vi "Scale Image - subvi.vi"(8 "Array Size":i32, 9 "99:1?":bool, 10 "Black/White Levels":cluster{ext, ext}(slide)={1.0, 65535.0} scale=-32768.0..32767.0, 11 "Image Array":i32[][](array[numeric])) -> (2 "Black/White Levels Out":cluster{ext, ext}(slide)={1.0, 65535.0} scale=-32768.0..32767.0, 3 "Image Array 2":i32[][](array[numeric]))   [LabVIEW 2014]
panel:
  out "Min":ext
  out "Max":ext
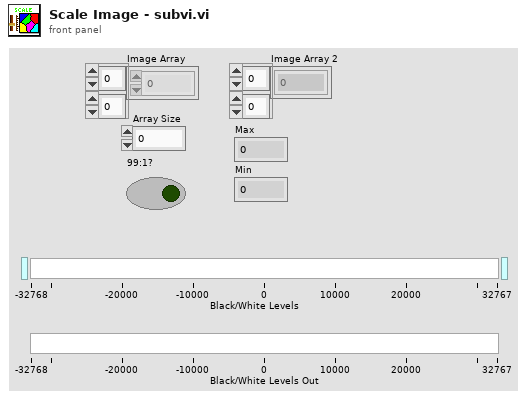
[diagram p1: front panel]
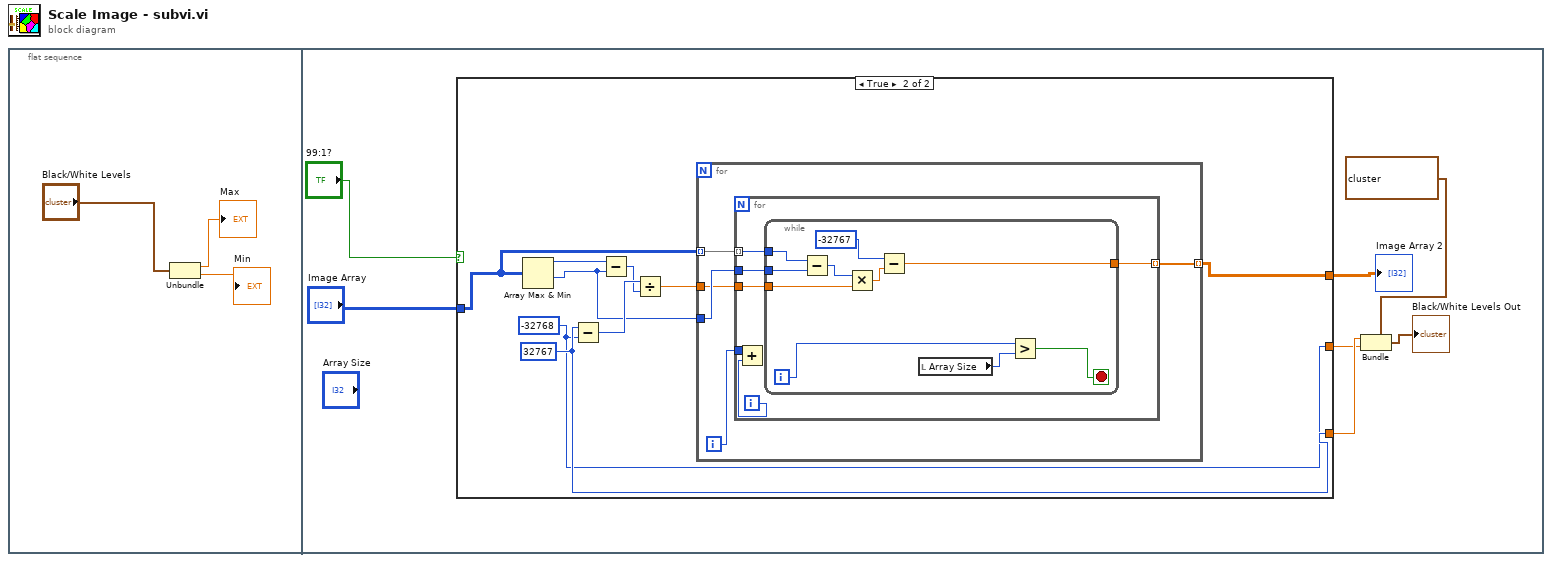
[diagram p0: block diagram]
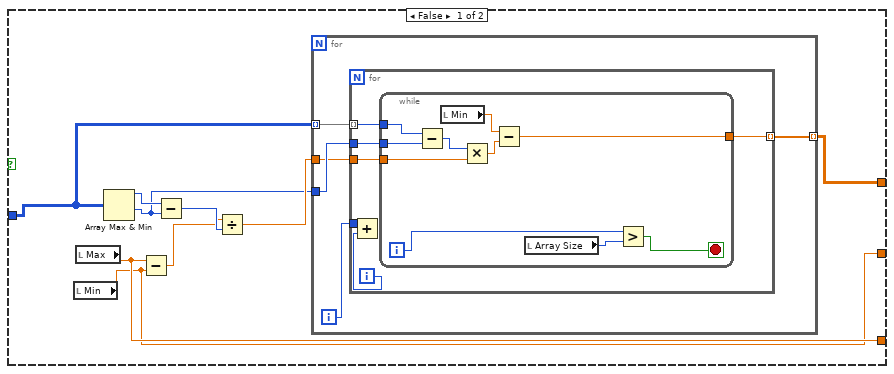
[diagram p2: hidden frame]
diagram:
  n1 = flat-sequence {
    frame #0 {
      n2 = Unbundle("Black/White Levels") -> (→"Max":ext, →"Min":ext)
    }
    frame #1 {
      n3 = case shown="True" "99:1?" {
        tunnel: "Image Array" -> [w16 w43]
        tunnel: [w14 w44] -> w10
        tunnel: [w12 w42] -> w5
        tunnel: [w11 w41] -> w4
        frame False {
          n4 = local read "Min"() -> (w11:ext)
          n5 = local read "Max"() -> (w12:ext)
          n6 = Array Max & Min(array=w16) -> (max value=w19:i32, min value=w13:i32)  [unwired: 2 out]
          n7 = Subtract(x=w12, y=w11) -> (x-y=w17:ext)
          n8 = Subtract(x=w19, y=w13) -> (x-y=w18:i32)
          n9 = Divide(x=w17, y=w18) -> (x/y=w15:ext)
          n10 = for {
            tunnel: w16 -> [w24] mode=indexing
            tunnel: w15 -> [w22]
            tunnel: w13 -> [w23]
            tunnel: [w20] -> w14 mode=indexing
            i -> [w21]
            n11 = for {
              tunnel: w24 -> [w30] mode=indexing
              tunnel: w23 -> [w29]
              tunnel: w22 -> [w28]
              tunnel: w21 -> [w27]
              tunnel: [w25] -> w20 mode=indexing
              i -> [w26]
              n12 = Add(x=w27, y=w26) -> ()  [unwired: 1 out]
              n13 = while {
                tunnel: w29 -> [w39]
                tunnel: w28 -> [w37]
                tunnel: w30 -> [w40]
                tunnel: [w35] -> w25
                i -> [w33]
                stop <- w31 stop-if-true
                n14 = Subtract(x=w40, y=w39) -> (x-y=w38:i32)
                n15 = local read "Min"() -> (w34:ext)
                n16 = Multiply(x=w38, y=w37) -> (x*y=w36:ext)
                n17 = Subtract(x=w34, y=w36) -> (x-y=w35:ext)
                n18 = local read "Array Size"() -> (w32:i32)
                n19 = Greater?(x=w33, y=w32) -> (0:w31:bool)
              }
            }
          }
        }
        frame True {
          w42 = 32767
          w41 = -32768
          n20 = Array Max & Min(array=w43) -> (max value=w49:i32, min value=w45:i32)  [unwired: 2 out]
          n21 = Subtract(x=w42, y=w41) -> (x-y=w48:i32)
          n22 = Subtract(x=w49, y=w45) -> (x-y=w47:i32)
          n23 = Divide(x=w48, y=w47) -> (x/y=w46:dbl)
          n24 = for {
            tunnel: w43 -> [w54] mode=indexing
            tunnel: w46 -> [w52]
            tunnel: w45 -> [w53]
            tunnel: [w50] -> w44 mode=indexing
            i -> [w51]
            n25 = for {
              tunnel: w54 -> [w60] mode=indexing
              tunnel: w53 -> [w59]
              tunnel: w52 -> [w58]
              tunnel: w51 -> [w57]
              tunnel: [w55] -> w50 mode=indexing
              i -> [w56]
              n26 = Add(x=w57, y=w56) -> ()  [unwired: 1 out]
              n27 = while {
                tunnel: w59 -> [w69]
                tunnel: w58 -> [w67]
                tunnel: w60 -> [w70]
                tunnel: [w64] -> w55
                i -> [w63]
                stop <- w61 stop-if-true
                n28 = Subtract(x=w70, y=w69) -> (x-y=w68:i32)
                n29 = Multiply(x=w68, y=w67) -> (x*y=w66:dbl)
                n30 = Subtract(x=-32767, y=w66) -> (x-y=w64:dbl)
                n31 = local read "Array Size"() -> (w62:i32)
                n32 = Greater?(x=w63, y=w62) -> (0:w61:bool)
              }
            }
          }
        }
      }
      "Image Array 2" <- w10
      n33 = Bundle(cluster=cluster{ext, ext} {140.1330472102979, 65535.0} ("Black/White Levels 2"), w5, w4) -> (→"Black/White Levels Out":cluster{ext, ext})
    }
  }
